vi "CLC_Switch_TRxMode_0200_0188.vi"(8 "error in (no error)":errorcluster, 11 "TCPIPin":T3={"address"="192.168.100.111", "remote port or service name"=5025, "timeout ms (60000)"=10000}) -> (0 "error out":errorcluster, 1 "OK?":bool, 3 "TCPIPin 2":T3={"address"="192.168.100.111", "remote port or service name"=5025, "timeout ms (60000)"=10000})   [LabVIEW 2023]
uses:
  CTL/0200_TDD.ctl
  CTL/0188_TDD.ctl
panel:
  in  "0188":T1
  in  "0200":T2
  out "data out":string
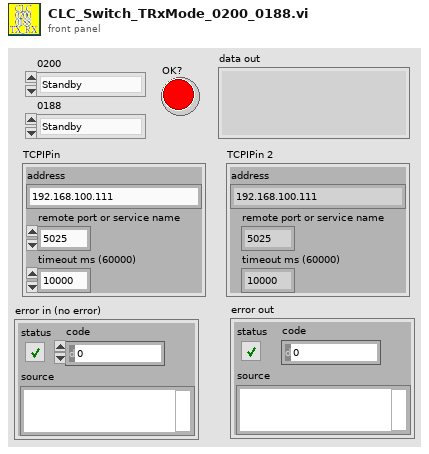
[diagram p1: front panel]
types:
  T1 = typedef "0188_TDD.ctl" = enum16{"Standby", "TX_LS", "RX_LS", "Sleep", "TX_HS", "RX_HS", "TX_ByPass", "RX_ByPass", "Loft_Cal_LS", "Loft_Cal_HS", "STandbyByPass"}
  T2 = typedef "0200_TDD.ctl" = enum16{"Standby", "TX", "RX", "Sleep"}
  T3 = cluster{"address":string, "remote port or service name":u16, "timeout ms (60000)":i32}
  T4 = enum16{"Standard", "Buffered", "CRLF", "Immediate"}
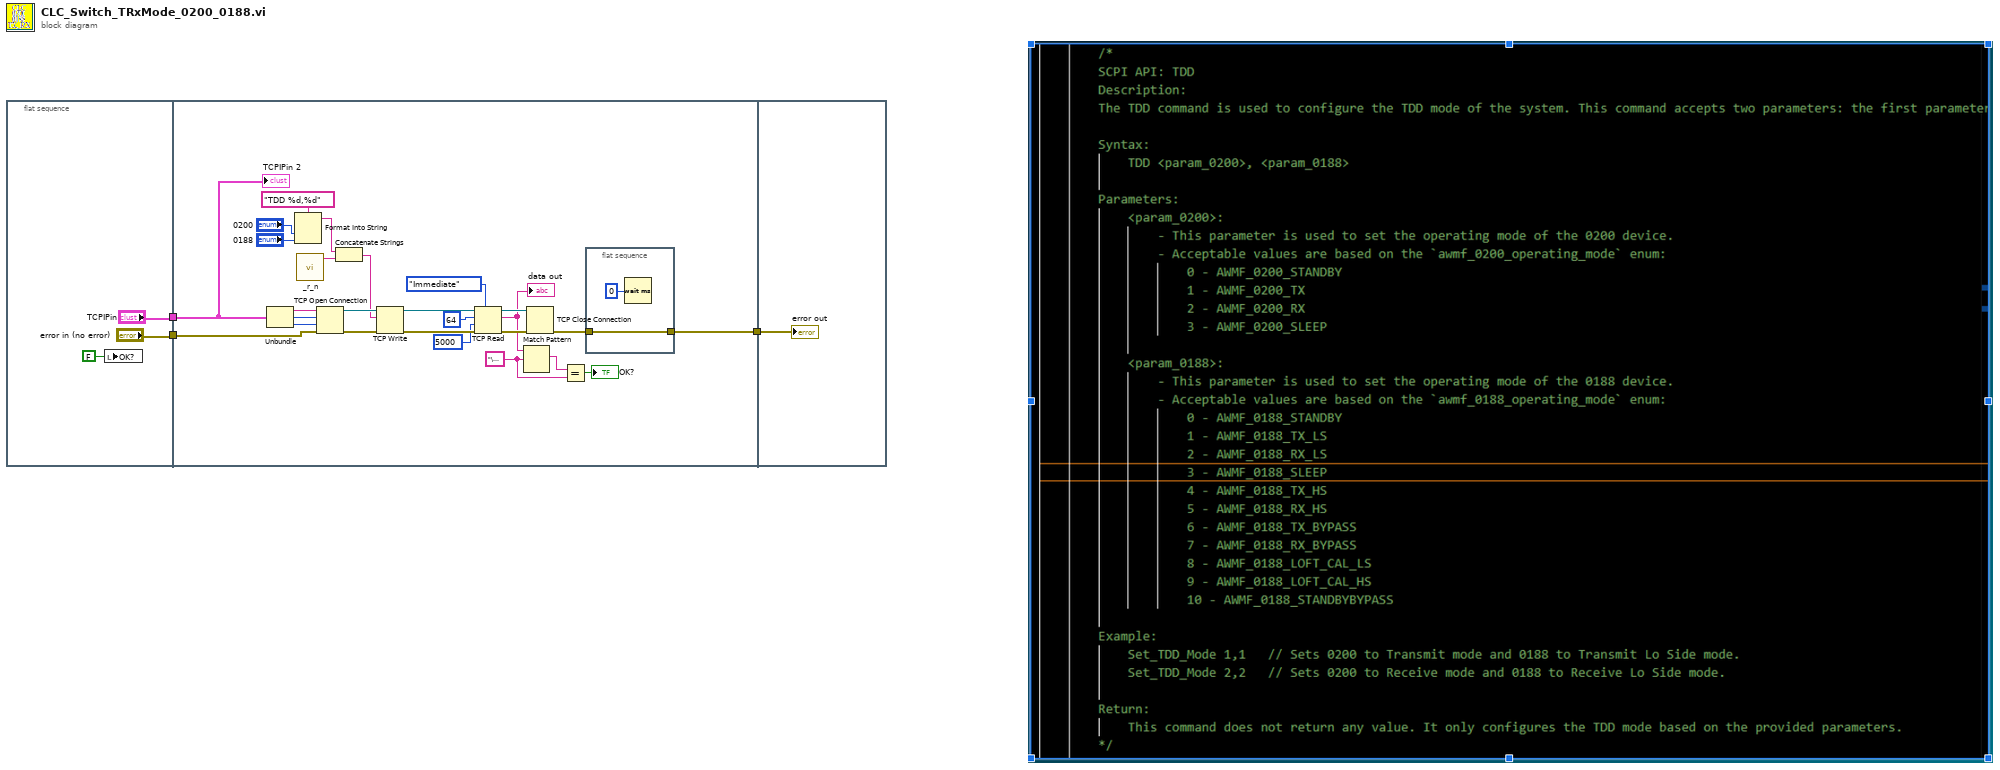
[diagram p0: block diagram]
diagram:
  n1 = flat-sequence {
    tunnel: ["TCPIPin"] -> w3
    tunnel: ["error in (no error)"] -> w2
    tunnel: w3 -> [w32]
    tunnel: w2 -> [w31]
    tunnel: [w10] -> w1
    tunnel: w1 -> [w35]
    frame #0 {
      n2 = local write "OK?"(FALSE ("OK?")) -> ()
    }
    frame #1 {
      w13 = "\u0000" ("string")
      n3 = Unbundle(w32) -> ("address"=w27:string, "remote port or service name"=w26:u16, "timeout ms (60000)"=w25:i32)
      n4 = Format Into String(format string="TDD %d,%d" ("data in"), "0200", "0188") -> (resulting string=w23:string)  [unwired: 2 in, 1 out]
      n5 = call "_r_n.vi"() -> ("command"=w9:string)  [unwired: 5 in]
      n6 = TCP Open Connection(address=w27, remote port or service name=w26, timeout ms (60000)=w25, error in (no error)=w31) -> (connection ID=w30:refnum<k5>, error out=w29:errorcluster)  [unwired: 1 in]
      n7 = Concatenate Strings(w23, w9) -> (w28:string)
      n8 = TCP Write(connection ID=w30, data in=w28, error in (no error)=w29) -> (connection ID out=w21:refnum<k5>, error out=w22:errorcluster)  [unwired: 1 in, 1 out]
      n9 = TCP Read(connection ID=w21, bytes to read=64, error in (no error)=w22, 7:T4."Immediate" ("mode (standard)"), 9:5000 ("timeout ms (25000)")) -> (connection ID out=w20:refnum<k5>, data out=w15:string, error out=w19:errorcluster)
      "data out" <- w15
      n10 = Match Pattern(string=w15, regular expression=w13) -> (match substring=w14:string)  [unwired: 1 in, 3 out]
      n11 = TCP Close Connection(connection ID=w20, error in (no error)=w19) -> (error out=w11:errorcluster)  [unwired: 1 in, 1 out]
      n12 = Equal?(x=w14, y=w13) -> (x = y?=→"OK?":bool)
      n13 = flat-sequence {
        tunnel: w11 -> [w34]
        tunnel: [w34] -> w10
        frame #0 {
          n14 = Wait (ms)(milliseconds to wait=u32 0) -> ()  [unwired: 1 out]
        }
      }
      "TCPIPin 2" <- w32
    }
    frame #2 {
      "error out" <- w35
    }
  }
